vi "Query with 1D Integer Result.vi"(8 "error in (no error)":errorcluster, 10 "Query string":string, 11 "AbstractHappyDatabase in":refnum<class "AbstractHappyDatabase.lvclass">) -> (0 "error out":errorcluster, 2 "Result":i32[](array[numeric]), 3 "AbstractHappyDatabase out":refnum<class "AbstractHappyDatabase.lvclass">)   [LabVIEW 2020, in "IDatabase.lvlib" / "AbstractHappyDatabase.lvclass"]
uses:
  AbstractHappyDatabase.lvclass
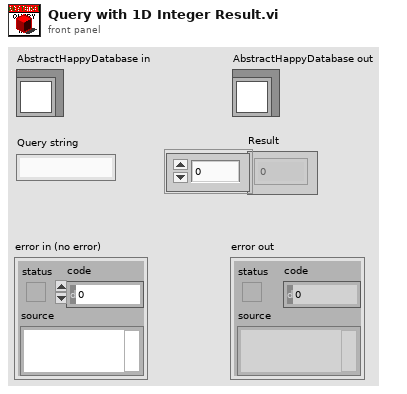
[diagram p1: front panel]
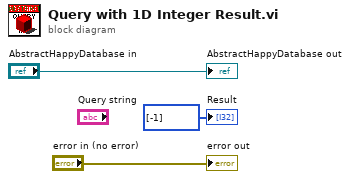
[diagram p0: block diagram]
diagram:
  "error out" <- "error in (no error)"
  "AbstractHappyDatabase out" <- "AbstractHappyDatabase in"
  "Result" <- i32[] [-1] ("Result")
